vi "GeoFonu_v1.vi"() -> ()   [LabVIEW 2014]
uses:
  <vilib>/Instr/_visa.llb/VISA Set IO Buffer Mask.ctl
  <vilib>/Instr/_visa.llb/VISA Flush IO Buffer Mask.ctl
  <vilib>/Instr/_visa.llb/VISA Configure Serial Port (Instr).vi
panel:
  out "Sensor3":i32[](graph)=[1413, 1176, 975, 827, 809, 872, 976, 1209, 1452, 1650, 1793, 1822, 1740, 1612, 1369, 1130, 938, 821, 809, 886, 1015, 1246, 1499, 1693, 1808, 1826, 1722, 1564, 1307, 1076, 901, 809, 823, 905, 1066, 1319, 1540, 1725, 1815, 1795, 1702, 1527, 1264, 1046, 874, 826, 853, 936, 1133, 1384, 1596, 1765, 1818, 1766, 1672, 1451, 1212, 1006, 848, 814, 867, 963, 1183, 1419, 1637, 1791, 1822, 1752, 1640, 1399, 1166, 964, 834, 815, 887, 996, 1240, 1474, 1673, 1805, 1827, 1747, 1612, 1356, 1122, 935, 828, 817, 897, 1033, 1287, 1520, 1714, 1815, 1815, 1725, 1564, 1305, 1077, 908, 822, 842, 925, 1093, 1345, 1568, 1759, 1814, 1784, 1697, 1514, 1253, 1045, 878, 827, 854, 944, 1141, 1393, 1614, 1790, 1860, 1818, 1702, 1473, 1230, 1016, 865, 834, 894, 997, 1228, 1459, 1664, 1810, 1834, 1750, 1628, 1377, 1147, 953, 827, 816, 892, 1022, 1301, 1523, 1723, 1826, 1822, 1733, 1576, 1316, 1093, 922, 837, 852, 930, 1089, 1340, 1557, 1741, 1822, 1809, 1717, 1533, 1270, 1050, 885, 838, 872, 957, 1154, 1407, 1622, 1789, 1832, 1779, 1698, 1465, 1212, 1012, 856, 821, 884, 983, 1213, 1456, 1660, 1805, 1834, 1754, 1638, 1391, 1146, 954, 829, 813, 892, 1016, 1266, 1493, 1687, 1807, 1821, 1733, 1589, 1333, 1101, 922, 820, 824, 906, 1051, 1314, 1539, 1728, 1847, 1823, 1735, 1547, 1282, 1065, 898, 830, 860, 941, 1127, 1377, 1584, 1764, 1828, 1783, 1689, 1486, 1228, 1030, 869, 841, 896, 983, 1205, 1444, 1657, 1818, 1847, 1783, 1670, 1423, 1183, 983, 850, 826, 895, 1008, 1241, 1473, 1707, 1831, 1841, 1756, 1615, 1354, 1115, 929, 824, 829, 917, 1054, 1306, 1528, 1726, 1821, 1808, 1718, 1557, 1293, 1066, 900, 825, 850, 929, 1100, 1352, 1569, 1748, 1824, 1773, 1698, 1502, 1250, 1037, 872, 830, 863, 953, 1156, 1400, 1623, 1792, 1833, 1780, 1683, 1451, 1216, 1016, 865, 845, 913, 1008, 1248, 1480, 1680, 1817, 1847, 1760, 1634, 1376, 1141, 953, 844, 835, 915, 1032, 1286, 1522, 1707, 1822, 1828, 1731, 1578, 1317, 1090, 912, 831, 839, 919, 1083, 1333, 1556, 1740, 1824, 1805, 1712, 1525, 1261, 1046, 884, 822, 848, 933, 1151, 1396, 1620, 1787, 1836, 1786, 1688, 1473, 1221, 1017, 862, 824, 886, 987, 1213, 1482, 1681, 1827, 1847, 1757, 1636, 1385, 1158, 970, 847, 832, 913, 1041, 1283, 1514, 1717, 1831, 1838, 1750, 1596, 1332, 1097, 925, 832, 848, 925, 1089, 1340, 1557, 1780, 1851, 1830, 1737, 1548, 1276, 1051, 886, 834, 865, 950, 1146, 1398, 1620, 1789, 1844, 1797, 1702, 1485, 1228, 1024, 872, 838, 887, 983, 1198, 1444, 1657, 1813, 1849, 1780, 1667, 1434, 1190, 990, 853, 830, 893, 1002, 1246, 1483, 1689, 1812, 1834, 1746, 1610, 1357, 1122, 942, 828, 830, 916, 1048, 1312, 1515, 1714, 1820, 1823, 1735, 1575, 1316, 1091, 915, 825, 850, 939, 1103, 1353, 1569, 1782, 1841, 1822, 1716, 1522, 1264, 1049, 881, 829, 867, 948, 1158, 1398, 1622, 1796, 1838, 1791, 1688, 1467, 1211, 1004, 855, 822, 884, 980, 1212, 1453, 1658, 1805, 1840, 1772, 1651, 1407, 1167, 980, 846, 833, 904, 1017, 1262, 1498, 1694, 1822, 1836, 1747, 1606, 1347, 1112, 933, 839, 838, 923, 1072, 1315, 1544, 1735, 1828, 1820, 1730, 1564, 1303, 1079, 907, 834, 859, 938, 1109, 1366, 1583, 1762, 1834, 1809, 1715, 1527, 1261, 1041, 879, 835, 874, 956, 1162, 1411, 1628, 1794, 1839, 1817, 1747, 1557, 1324, 1137, 997, 975, 1035, 1144, 1376, 1627, 1839, 1992, 2010, 1954, 1831, 1585, 1340, 1150, 1021, 1005, 1081, 1207, 1451, 1689, 1881, 2005, 2018, 1941, 1797, 1537, 1299, 1120, 1011, 1012, 1088, 1241, 1498, 1731, 1918, 2027, 1999, 1913, 1747, 1482, 1259, 1080, 1008, 1025, 1108, 1282, 1541, 1772, 1949, 2014, 1983, 1897, 1697, 1440, 1224, 1056, 1006, 1049, 1137, 1340, 1592, 1808, 1980, 2012, 1967, 1867, 1639, 1380, 1178, 1023, 995, 1050, 1151, 1382, 1631, 1836, 1989, 2018, 1952, 1828, 1581, 1335, 1153, 1023, 1008, 1075, 1203, 1444, 1686, 1880, 1998, 2018, 1942, 1795, 1536, 1298, 1112, 1005, 1006, 1087, 1245, 1493, 1725, 1913, 2005, 1992, 1909, 1735, 1468, 1237, 1076, 995, 1017, 1130, 1307, 1560, 1778, 1946, 2005, 1971, 1893, 1678, 1427, 1209, 1045, 996, 1037, 1131, 1338, 1583, 1802, 1967, 2004, 1952, 1847, 1614, 1361, 1160, 1012, 983, 1048, 1156, 1399, 1641, 1841, 1991, 2012, 1941, 1799, 1559, 1331, 1137, 1006, 995, 1075, 1209, 1460, 1697, 1886, 1999, 2004, 1923, 1769, 1509, 1275, 1088, 998, 1012, 1090, 1248, 1498, 1734, 1919, 2000, 1992, 1908, 1725, 1471, 1232, 1063, 1001, 1025, 1108, 1293, 1551, 1773, 1954, 2011, 1976, 1880, 1668, 1422, 1203, 1049, 1005, 1052, 1141, 1365, 1618, 1832, 1991, 2018, 1963, 1849, 1604, 1359, 1161, 1014, 988, 1053, 1172, 1412, 1656, 1857, 1989, 2014, 1938, 1805, 1551, 1306, 1120, 1004, 990, 1066, 1204, 1458, 1702, 1892, 1992, 1997, 1912, 1746, 1491, 1262, 1082, 996, 1012, 1087, 1246, 1519, 1741, 1925, 1997, 1983, 1896, 1706, 1448, 1224, 1059, 996, 1023, 1112, 1301, 1554, 1780, 1959, 2005, 1978, 1867, 1651, 1398, 1190, 1022, 1003, 1054, 1154, 1382, 1620, 1826, 1986, 2013, 1948, 1827, 1586, 1339, 1148, 1004, 985, 1062, 1180, 1425, 1667, 1855, 1990, 1994, 1913, 1773, 1517, 1285, 1103, 998, 994, 1082, 1217, 1499, 1730, 1915, 2001, 1991, 1902, 1728, 1475, 1240, 1067, 1003, 1030, 1112, 1294, 1552, 1776, 1950, 1997, 1962, 1867, 1644, 1408, 1190, 1029, 988, 1034, 1116, 1340, 1582, 1797, 1970, 2006, 1954, 1841, 1598, 1354, 1154, 1001, 979, 1048, 1159, 1393, 1640, 1836, 1984, 2025, 1950, 1807, 1544, 1307, 1112, 995, 981, 1059, 1203, 1462, 1702, 1886, 1988, 1983, 1905, 1738, 1480, 1251, 1075, 990, 1008, 1088, 1257, 1511, 1737, 1918, 1991, 1975, 1894, 1699, 1442, 1216, 1052, 999, 1038, 1115, 1323, 1570, 1791, 1960, 1999, 1950, 1852, 1627, 1385, 1174, 1020, 988, 1041, 1146, 1378, 1620, 1831, 1983, 2005, 1941, 1822, 1570, 1334, 1132, 999, 990, 1051, 1178, 1420, 1664, 1855, 1976, 1983, 1909, 1768, 1515, 1275, 1100, 1008, 991, 1071, 1215, 1469, 1707, 1896, 1988, 1981, 1896, 1728, 1472, 1256, 1072, 1008, 1029, 1108, 1305, 1544, 1782, 1946, 1996, 1957, 1862, 1642, 1396, 1189, 1022, 993, 1048, 1155, 1377, 1625, 1828, 1976, 2001, 1934, 1808, 1554, 1311, 1120, 996, 979, 1049, 1180, 1425, 1659, 1854, 1975, 1985, 1925, 1769, 1507, 1267, 1083, 988, 1001, 1082, 1238, 1496, 1731, 1911, 1991, 1969, 1883, 1702, 1439, 1212, 1039, 975, 1002, 1092, 1282, 1538, 1757, 1930, 1986, 1952, 1856, 1648, 1398, 1184, 1018, 977, 1022, 1144, 1367, 1612, 1822, 1973, 2004, 1944, 1826, 1581, 1339, 1148, 996, 979, 1051, 1162, 1407, 1652, 1847, 1976, 2000, 1921, 1786, 1531, 1286, 1100, 987, 975, 1067, 1204, 1461, 1692, 1889, 1987, 1982, 1901, 1738, 1477, 1241, 1074, 982, 1005, 1081, 1250, 1502, 1731, 1909, 1983, 1963, 1877, 1694, 1432, 1204, 1054, 998, 1035, 1124, 1322, 1573, 1784, 1958, 1998, 1955, 1851, 1631, 1388, 1178, 1029, 990, 1049, 1153, 1384, 1634, 1834, 1983, 2005]
  out "Sensor2":i32[](graph)=[862, 673, 556, 495, 533, 632, 742, 958, 1142, 1263, 1327, 1282, 1170, 1050, 830, 650, 534, 487, 547, 664, 788, 1007, 1178, 1293, 1320, 1272, 1160, 1006, 784, 622, 526, 503, 569, 682, 837, 1053, 1202, 1301, 1311, 1243, 1137, 969, 746, 597, 510, 534, 605, 701, 885, 1091, 1233, 1322, 1294, 1211, 1106, 909, 712, 572, 490, 523, 617, 722, 926, 1118, 1245, 1327, 1286, 1182, 1068, 856, 676, 553, 493, 541, 651, 771, 990, 1172, 1281, 1324, 1289, 1177, 1039, 819, 647, 543, 502, 553, 660, 796, 1021, 1194, 1306, 1324, 1262, 1149, 996, 774, 622, 531, 514, 576, 684, 850, 1064, 1228, 1307, 1309, 1235, 1132, 966, 744, 602, 518, 531, 608, 713, 892, 1095, 1243, 1331, 1343, 1237, 1119, 904, 723, 590, 503, 548, 648, 759, 967, 1144, 1276, 1334, 1287, 1180, 1057, 834, 660, 545, 495, 548, 660, 781, 1040, 1199, 1318, 1325, 1274, 1152, 1011, 784, 626, 536, 527, 580, 689, 838, 1048, 1202, 1310, 1319, 1244, 1140, 968, 741, 588, 510, 542, 620, 720, 902, 1105, 1245, 1327, 1295, 1217, 1129, 908, 719, 576, 505, 547, 639, 736, 958, 1144, 1270, 1344, 1294, 1182, 1058, 838, 659, 543, 497, 542, 655, 780, 1008, 1183, 1288, 1329, 1274, 1168, 1025, 805, 643, 543, 493, 576, 684, 822, 1044, 1202, 1311, 1351, 1265, 1147, 971, 754, 612, 512, 518, 589, 708, 880, 1088, 1233, 1327, 1307, 1224, 1127, 938, 734, 599, 510, 556, 638, 747, 942, 1143, 1263, 1348, 1315, 1210, 1089, 869, 690, 564, 502, 548, 650, 772, 977, 1149, 1307, 1344, 1293, 1188, 1038, 817, 651, 537, 508, 564, 683, 824, 1037, 1194, 1295, 1315, 1247, 1140, 991, 767, 610, 518, 519, 584, 687, 852, 1070, 1219, 1312, 1307, 1228, 1124, 958, 743, 601, 514, 535, 612, 718, 907, 1108, 1249, 1340, 1310, 1225, 1118, 910, 713, 589, 510, 558, 652, 767, 987, 1164, 1286, 1341, 1305, 1193, 1059, 828, 664, 556, 519, 562, 677, 808, 1027, 1193, 1299, 1332, 1281, 1167, 1019, 791, 627, 534, 518, 584, 687, 834, 1060, 1219, 1311, 1319, 1248, 1137, 963, 748, 599, 512, 527, 605, 705, 913, 1104, 1252, 1328, 1319, 1218, 1108, 912, 718, 580, 502, 537, 632, 755, 961, 1174, 1290, 1349, 1303, 1185, 1066, 842, 664, 551, 502, 560, 671, 796, 1019, 1186, 1303, 1343, 1291, 1177, 1027, 800, 629, 537, 524, 589, 689, 843, 1063, 1216, 1351, 1346, 1260, 1157, 972, 761, 610, 516, 533, 603, 707, 891, 1099, 1251, 1339, 1312, 1221, 1124, 921, 717, 588, 514, 543, 635, 736, 945, 1140, 1271, 1344, 1307, 1209, 1099, 877, 686, 564, 506, 545, 648, 762, 978, 1165, 1281, 1338, 1291, 1177, 1046, 821, 660, 531, 511, 560, 670, 804, 1032, 1185, 1292, 1332, 1276, 1159, 1006, 792, 631, 537, 518, 589, 688, 854, 1064, 1217, 1340, 1328, 1242, 1132, 948, 736, 601, 514, 532, 618, 716, 910, 1103, 1253, 1340, 1315, 1232, 1125, 911, 709, 585, 498, 535, 631, 747, 950, 1141, 1269, 1335, 1292, 1199, 1076, 861, 685, 564, 511, 559, 661, 777, 999, 1176, 1291, 1337, 1285, 1174, 1040, 817, 638, 547, 515, 569, 684, 829, 1041, 1207, 1311, 1332, 1269, 1153, 1000, 775, 624, 526, 520, 588, 681, 855, 1073, 1228, 1328, 1327, 1247, 1135, 963, 745, 608, 514, 531, 617, 718, 912, 1115, 1249, 1340, 1311, 1242, 1177, 991, 811, 693, 615, 654, 756, 859, 1074, 1266, 1392, 1460, 1409, 1306, 1197, 975, 800, 686, 621, 671, 776, 892, 1121, 1284, 1399, 1453, 1409, 1290, 1151, 933, 754, 664, 626, 680, 788, 930, 1164, 1315, 1422, 1448, 1386, 1267, 1109, 887, 738, 648, 636, 714, 811, 985, 1198, 1345, 1441, 1432, 1353, 1245, 1070, 855, 722, 623, 654, 726, 836, 1025, 1225, 1370, 1460, 1415, 1338, 1228, 1026, 824, 695, 622, 658, 756, 852, 1062, 1249, 1382, 1462, 1410, 1305, 1184, 966, 790, 673, 625, 671, 779, 897, 1117, 1290, 1399, 1447, 1404, 1294, 1154, 928, 761, 655, 639, 689, 789, 944, 1161, 1322, 1421, 1443, 1375, 1259, 1095, 872, 724, 633, 634, 705, 838, 1002, 1209, 1344, 1441, 1433, 1341, 1241, 1055, 839, 708, 624, 638, 720, 835, 1027, 1224, 1357, 1441, 1404, 1324, 1213, 1006, 813, 682, 614, 648, 759, 872, 1087, 1264, 1382, 1447, 1412, 1304, 1174, 962, 790, 676, 614, 670, 774, 909, 1134, 1286, 1412, 1443, 1394, 1274, 1138, 916, 753, 653, 629, 696, 797, 951, 1158, 1315, 1420, 1441, 1366, 1255, 1090, 876, 718, 629, 639, 710, 796, 987, 1199, 1353, 1445, 1427, 1341, 1232, 1054, 849, 705, 635, 658, 738, 834, 1044, 1242, 1378, 1461, 1415, 1322, 1209, 985, 792, 680, 611, 650, 759, 882, 1098, 1280, 1395, 1448, 1407, 1302, 1163, 948, 771, 655, 619, 668, 772, 909, 1124, 1302, 1407, 1441, 1388, 1274, 1116, 901, 747, 643, 634, 698, 801, 958, 1176, 1331, 1423, 1428, 1353, 1248, 1079, 859, 709, 628, 637, 711, 823, 995, 1212, 1357, 1452, 1428, 1349, 1235, 1037, 835, 702, 613, 654, 749, 849, 1062, 1246, 1364, 1450, 1411, 1311, 1187, 973, 796, 670, 605, 646, 763, 885, 1105, 1282, 1399, 1441, 1386, 1270, 1138, 910, 751, 642, 627, 682, 788, 927, 1166, 1322, 1427, 1442, 1375, 1261, 1104, 896, 734, 634, 638, 710, 807, 982, 1204, 1341, 1436, 1419, 1333, 1225, 1032, 839, 698, 613, 644, 727, 821, 1033, 1234, 1367, 1453, 1415, 1311, 1195, 981, 801, 676, 601, 658, 757, 874, 1079, 1257, 1378, 1450, 1427, 1306, 1174, 942, 770, 663, 614, 656, 771, 908, 1135, 1306, 1404, 1428, 1376, 1260, 1099, 888, 725, 635, 627, 690, 805, 954, 1170, 1328, 1427, 1423, 1348, 1241, 1075, 860, 708, 626, 641, 722, 821, 1012, 1220, 1359, 1439, 1417, 1322, 1224, 1013, 826, 683, 606, 640, 737, 842, 1055, 1240, 1376, 1448, 1401, 1295, 1181, 962, 786, 663, 603, 654, 755, 880, 1101, 1275, 1391, 1436, 1385, 1274, 1139, 915, 750, 643, 614, 669, 776, 913, 1137, 1299, 1415, 1438, 1369, 1257, 1098, 883, 741, 637, 638, 713, 817, 999, 1211, 1355, 1427, 1418, 1336, 1223, 1022, 840, 699, 613, 653, 746, 858, 1066, 1246, 1382, 1438, 1412, 1301, 1178, 954, 774, 655, 610, 651, 753, 888, 1104, 1277, 1391, 1428, 1380, 1288, 1136, 906, 738, 639, 621, 688, 785, 935, 1153, 1318, 1414, 1420, 1349, 1244, 1074, 855, 709, 616, 627, 693, 810, 983, 1192, 1335, 1423, 1415, 1329, 1230, 1032, 838, 696, 606, 642, 726, 857, 1052, 1240, 1373, 1444, 1396, 1307, 1184, 967, 792, 672, 605, 652, 759, 862, 1087, 1268, 1379, 1435, 1398, 1286, 1144, 930, 751, 642, 614, 659, 773, 917, 1141, 1299, 1410, 1425, 1362, 1264, 1106, 887, 726, 630, 618, 681, 789, 950, 1163, 1314, 1408, 1411, 1334, 1237, 1066, 841, 705, 623, 643, 723, 829, 1018, 1220, 1357, 1444, 1407, 1325, 1216, 1021, 830, 693, 618, 642, 742, 845, 1064, 1244, 1376, 1447, 1407]
  out "Sensor1":i32[](graph)=[3, 2, 3, 3, 3, 0, 4, 5, 1, 1, 4, 2, 2, 1, 0, 4, 2, 2, 0, 1, 2, 3, 1, 3, 4, 1, 1, 4, 3, 0, 3, 2, 4, 3, 3, 1, 2, 2, 3, 2, 1, 3, 4, 3, 1, 3, 0, 4, 4, 2, 2, 0, 2, 4, 4, 2, 3, 2, 2, 4, 2, 0, 4, 4, 2, 2, 2, 2, 2, 2, 1, 4, 0, 1, 3, 3, 1, 3, 4, 2, 1, 3, 4, 2, 2, 3, 2, 0, 4, 4, 3, 3, 1, 2, 4, 4, 4, 0, 2, 17, 2, 4, 2, 3, 2, 3, 2, 2, 4, 4, 3, 4, 1, 0, 1, 0, 3, 4, 4, 3, 0, 3, 2, 3, 5, 1, 0, 2, 1, 0, 3, 2, 1, 3, 2, 4, 2, 0, 0, 2, 2, 2, 1, 0, 4, 1, 4, 1, 4, 3, 2, 1, 2, 4, 0, 29, 2, 1, 2, 2, 8, 1, 3, 4, 2, 2, 13, 2, 1, 0, 1, 1, 4, 3, 2, 4, 2, 1, 4, 5, 1, 4, 3, 1, 0, 2, 1, 4, 3, 0, 2, 4, 2, 2, 4, 2, 1, 2, 3, 3, 11, 1, 4, 4, 2, 4, 2, 3, 1, 1, 2, 3, 3, 4, 3, 0, 1, 2, 2, 5, 21, 4, 1, 2, 4, 2, 1, 3, 2, 3, 3, 0, 4, 3, 1, 3, 1, 4, 1, 3, 1, 5, 1, 4, 1, 3, 0, 3, 5, 3, 2, 2, 1, 4, 3, 2, 2, 4, 2, 3, 2, 1, 0, 1, 0, 3, 4, 6, 0, 4, 2, 2, 4, 2, 4, 4, 4, 2, 2, 1, 4, 2, 3, 3, 4, 4, 2, 0, 0, 0, 1, 3, 3, 2, 3, 1, 3, 2, 1, 1, 4, 6, 4, 1, 2, 10, 3, 4, 2, 3, 3, 3, 1, 3, 1, 3, 2, 4, 1, 4, 0, 2, 1, 4, 0, 0, 1, 3, 3, 4, 4, 0, 4, 3, 3, 8, 0, 2, 3, 1, 2, 1, 2, 4, 1, 3, 7, 4, 1, 3, 0, 1, 2, 3, 2, 1, 4, 4, 3, 4, 2, 4, 2, 4, 4, 1, 1, 1, 0, 4, 4, 1, 2, 4, 7, 4, 0, 1, 4, 1, 0, 11, 3, 3, 4, 2, 5, 4, 3, 4, 1, 5, 3, 3, 4, 1, 9, 4, 1, 2, 1, 4, 4, 3, 4, 1, 4, 2, 4, 4, 2, 2, 1, 2, 0, 1, 0, 5, 4, 2, 4, 3, 3, 4, 0, 3, 1, 2, 2, 5, 1, 4, 0, 0, 5, 3, 2, 3, 4, 5, 0, 2, 1, 2, 0, 2, 2, 4, 1, 4, 4, 3, 3, 2, 2, 6, 4, 3, 3, 3, 2, 3, 2, 4, 4, 2, 2, 4, 4, 2, 0, 1, 4, 1, 2, 3, 5, 1, 3, 1, 3, 1, 4, 4, 1, 4, 3, 2, 3, 2, 3, 2, 4, 2, 1, 4, 4, 3, 5, 1, 0, 0, 5, 13, 1, 4, 2, 2, 3, 4, 1, 4, 1, 1, 2, 1, 3, 2, 3, 4, 3, 3, 4, 1, 2, 4, 2, 3, 2, 2, 4, 5, 1, 1, 1, 4, 13, 1, 1, 1, 4, 1, 0, 2, 1, 1, 4, 2, 3, 0, 0, 0, 1, 0, 4, 0, 0, 0, 0, 0, 0, 0, 2, 0, 0, 3, 1, 1, 2, 0, 2, 2, 1, 2, 0, 3, 1, 2, 2, 1, 2, 3, 1, 4, 0, 4, 1, 2, 2, 4, 1, 2, 0, 4, 1, 3, 2, 3, 0, 3, 3, 2, 4, 4, 4, 4, 3, 2, 9, 4, 1, 0, 1, 4, 4, 1, 3, 4, 3, 0, 3, 5, 0, 3, 2, 0, 4, 2, 4, 1, 1, 4, 4, 2, 4, 4, 2, 3, 3, 3, 4, 0, 1, 2, 3, 3, 3, 2, 2, 4, 3, 3, 1, 8, 1, 0, 4, 4, 4, 0, 2, 4, 4, 0, 1, 3, 4, 1, 4, 3, 2, 3, 4, 5, 0, 3, 4, 3, 3, 4, 2, 1, 2, 2, 4, 2, 4, 3, 1, 0, 2, 4, 3, 4, 1, 4, 3, 3, 2, 4, 1, 3, 4, 1, 1, 3, 2, 3, 4, 1, 0, 4, 4, 2, 1, 3, 3, 3, 4, 3, 4, 1, 4, 1, 4, 4, 3, 0, 2, 2, 2, 1, 2, 0, 1, 2, 0, 4, 2, 6, 3, 2, 4, 5, 4, 1, 4, 3, 4, 2, 4, 3, 3, 3, 1, 4, 3, 2, 4, 2, 1, 4, 2, 3, 1, 4, 1, 2, 1, 1, 1, 4, 0, 2, 2, 1, 4, 4, 2, 2, 0, 2, 3, 3, 2, 4, 1, 3, 0, 3, 3, 4, 3, 2, 3, 2, 4, 2, 4, 3, 0, 4, 0, 3, 4, 1, 4, 1, 1, 0, 3, 3, 1, 4, 4, 3, 4, 5, 0, 2, 3, 4, 2, 3, 4, 3, 5, 3, 1, 4, 2, 4, 1, 1, 0, 3, 3, 2, 2, 4, 2, 4, 2, 4, 3, 4, 1, 1, 2, 4, 3, 3, 3, 2, 1, 3, 3, 4, 4, 4, 4, 5, 1, 4, 2, 1, 2, 4, 4, 1, 3, 2, 3, 2, 4, 0, 3, 2, 1, 0, 2, 0, 4, 1, 2, 4, 0, 3, 1, 5, 0, 3, 1, 2, 4, 4, 2, 1, 1, 4, 2, 0, 2, 3, 1, 4, 5, 3, 4, 2, 1, 0, 1, 1, 4, 0, 0, 4, 1, 3, 4, 4, 7, 0, 1, 2, 0, 2, 4, 4, 2, 3, 3, 2, 3, 2, 1, 3, 0, 2, 4, 2, 2, 5, 1, 4, 3, 2, 2, 2, 3, 2, 1, 2, 2, 3, 2, 5, 2, 3, 3, 2, 4, 2, 4, 8, 4, 2, 4, 4, 0, 4, 2, 4, 1, 4, 1, 4, 2, 4, 4, 2, 5, 3, 9, 1, 3, 3, 2, 4, 8, 2, 4, 4, 3, 2, 5, 1, 1, 2, 4, 3, 4, 4, 2, 3, 4, 3, 4, 1, 2, 4, 1, 2, 1, 0, 4, 2, 7, 4, 4, 4, 2, 1, 3, 2, 2, 2, 6, 4, 0, 2, 4, 2, 4, 4, 4, 3, 4, 0, 16, 1, 4, 5, 3, 2, 1, 4, 1, 1, 0, 3, 4, 3, 1, 4, 3, 2, 2, 1, 4, 2, 1, 3, 2, 3, 1, 4, 3, 1, 4, 0, 3, 2, 2, 3, 5, 4, 0, 4, 1, 3, 1, 4, 1, 2, 4, 17, 4, 1, 4, 3, 4, 2, 1, 4, 4, 4, 5, 4, 4, 4, 1, 4, 6, 2, 8, 3, 1, 3, 4, 4, 4, 2, 1, 2, 3, 0, 0, 3, 4, 4, 4, 4, 5, 3, 1, 4]
  in  "milliseconds to wait":u32=500
  in  "stop":bool
  in  "VISA resource name":refnum<visa-resource-name>
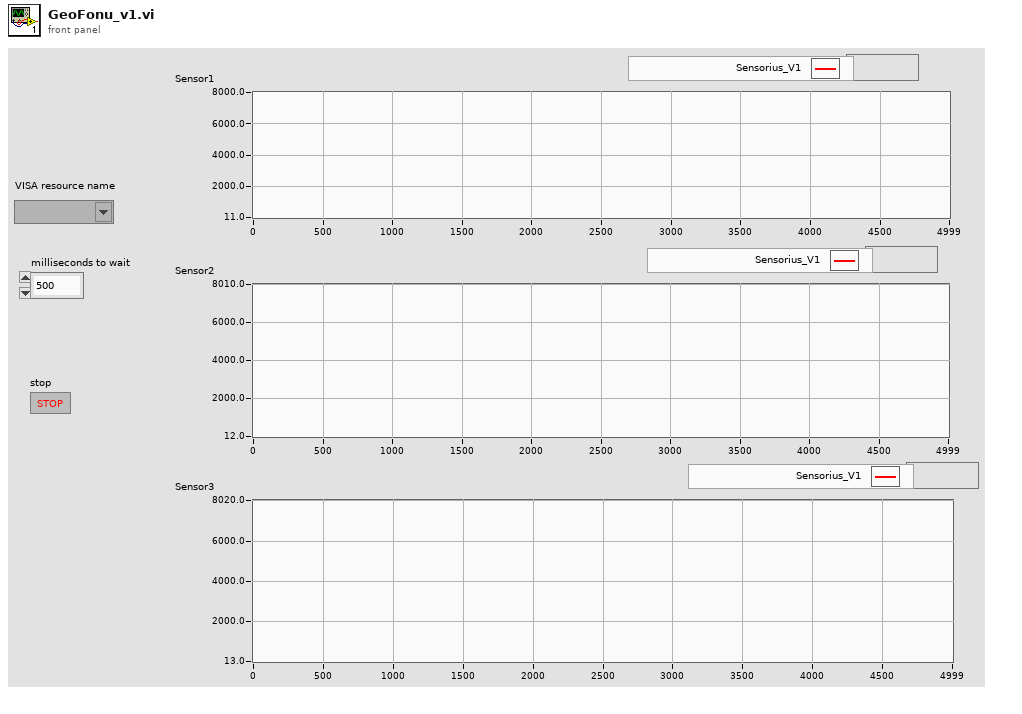
[diagram p1: front panel]
types:
  T1 = typedef "VISA Set IO Buffer Mask.ctl" = u16
  T2 = typedef "VISA Flush IO Buffer Mask.ctl" = u16
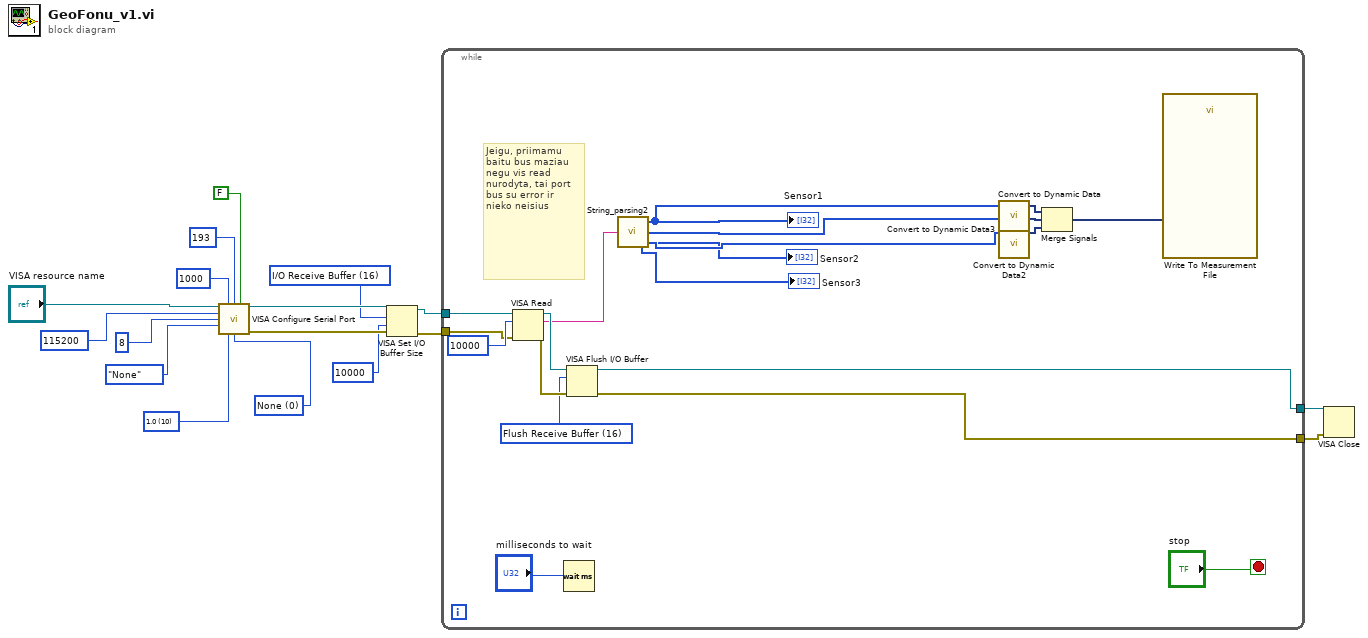
[diagram p0: block diagram]
diagram:
  w7 = T1 16 items=["I/O Receive Buffer"=16, "I/O Transmit Buffer"=32, "I/O Receive and Transmit Buffer"=48] ("Mask")
  w13 = u16 0 items=["None", "XON/XOFF", "RTS/CTS", "XON/XOFF & RTS/CTS", "DTR/DSR", "XON/XOFF & DTR/DSR"] ("flow control (0:none)")
  w14 = u16 10 items=["1.0"=10, "1.5"=15, "2.0"=20] ("stop bits (10: 1 bit)")
  n1 = call-poly "VISA Configure Serial Port"("VISA resource name"="VISA resource name", "timeout (10sec)"=u32 1000, "termination char\n(0xA = '\\n' = LF)"=u8 193 ("termination char\n(0xA = '\\n' = LF)"), "Enable Termination\nChar (T)"=FALSE ("Enable Termination\nChar (T)"), "baud rate (9600)"=u32 115200, "data bits (8)"=u16 8, "parity (0:none)"=enum16{"None", "Odd", "Even", "Mark", "Space"}."None", "stop bits (10: 1 bit)"=w14, "flow control (0:none)"=w13) -> ("VISA resource name out"=w9:refnum<visa-resource-name>, "error out"=w10:errorcluster)  [unwired: 5 in]
  n2 = VISA Set I/O Buffer Size(VISA resource name=w9, mask (16)=w7, size (4096)=u32 10000, error in (no error)=w10) -> (VISA resource name out=w3:refnum<visa-resource-name>, error out=w6:errorcluster)
  n3 = while {
    tunnel: w3 -> [w35]
    tunnel: w6 -> [w32]
    tunnel: [w26] -> w2
    tunnel: [w25] -> w1
    stop <- "stop" stop-if-true
    w29 = T2 16 items=["Flush Receive Buffer"=16, "Write Transmit Buffer to Device"=32, "Flush Receive Buffer (No I/O)"=64, "Flush Transmit Buffer"=128] ("Mask")
    # "Jeigu, priimamu baitu bus maziau negu vis read nurodyta, tai port bus su error ir nieko neisius"
    n4 = VISA Read(VISA resource name=w35, byte count=u32 10000, error in (no error)=w32) -> (VISA resource name out=w31:refnum<visa-resource-name>, read buffer=w27:string, error out=w30:errorcluster)  [unwired: 1 out]
    n5 = Wait (ms)(milliseconds to wait="milliseconds to wait") -> ()  [unwired: 1 out]
    n6 = VISA Flush I/O Buffer(VISA resource name=w31, mask (16)=w29, error in (no error)=w30) -> (VISA resource name out=w26:refnum<visa-resource-name>, error out=w25:errorcluster)
    n7 = call "String_parsing2.vi"("input string"=w27) -> ("V3"=w21:i32[], "V2"=w19:i32[], "V1"=w24:i32[])  [unwired: 2 in]
    "Sensor1" <- w24
    "Sensor2" <- w19
    "Sensor3" <- w21
    n8 = call "Convert to Dynamic Data"("Array"=w24) -> ("Dynamic Data Type"=w23:dynamicdata)  [unwired: 3 in]
    n9 = call "Convert to Dynamic Data3"("Array"=w19) -> ("Dynamic Data Type"=w18:dynamicdata)  [unwired: 3 in]
    n10 = call "Convert to Dynamic Data2"("Array"=w21) -> ("Dynamic Data Type"=w20:dynamicdata)  [unwired: 3 in]
    n11 = Merge Signals(w23, w18, w20) -> (w22:dynamicdata)
    n12 = call "Write To Measurement File"("Signals"=w22) -> ()  [unwired: 16 in, 3 out]
  }
  n13 = VISA Close(VISA resource name=w2, error in (no error)=w1) -> ()  [unwired: 1 out]
